vi "Pop.vi"(8 "error in (no error)":errorcluster, 11 "Signaller in":refnum<class "Signaller.lvclass">) -> (0 "error out":errorcluster, 2 "Has signal":bool, 3 "Signaller out":refnum<class "Signaller.lvclass">)   [LabVIEW 2018, in "Signaller.lvclass"]
uses:
  Signaller.lvclass
  Signaller.lvclass/Signaller.ctl
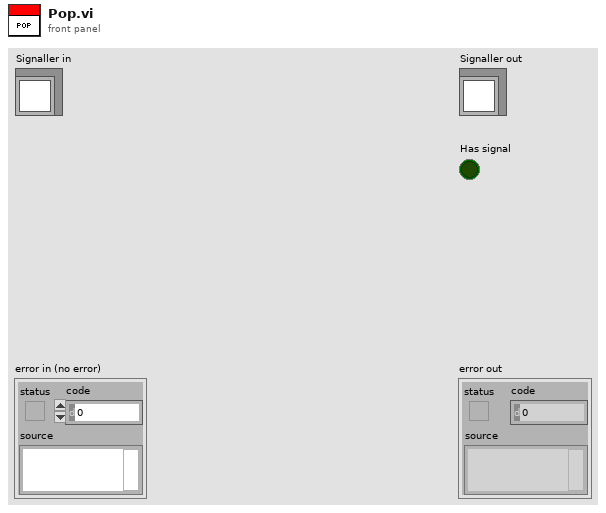
[diagram p1: front panel]
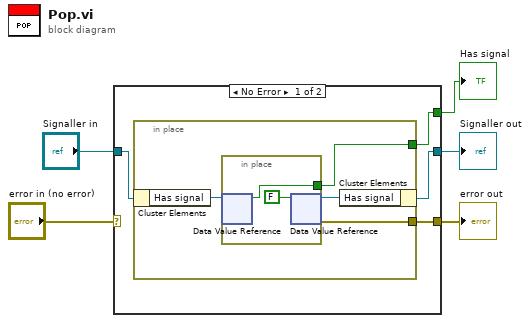
[diagram p0: block diagram]
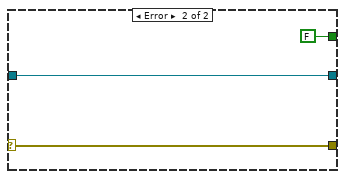
[diagram p2: hidden frame]
diagram:
  n1 = case shown="No Error" "error in (no error)" {
    selector: "error in (no error)" -> [_ w17]
    tunnel: [w6 w17] -> w4
    tunnel: [w8 w18] -> w2
    tunnel: "Signaller in" -> [w9 w18]
    tunnel: [w7 FALSE ("Has signal")] -> w1
    frame No Error {
      n2 = in-place {
        in-place-border: [w12] -> w7
        in-place-border: [w11] -> w6
        n3 = in-place-cluster #1(w9) -> ("Has signal"=w13:refnum<data-value>)
        n4 = in-place {
          in-place-border: [w14] -> w12
          n5 = in-place-dvr #2(w13) -> (w14:bool)  [unwired: 1 out]
          n6 = in-place-dvr #2(FALSE ("data value")) -> (w10:refnum<data-value>, w11:errorcluster)
        }
        n7 = in-place-cluster #1("Has signal"=w10) -> (w8:refnum<class "Signaller.lvclass">)
      }
    }
    frame Error {
    }
  }
  "error out" <- w4
  "Signaller out" <- w2
  "Has signal" <- w1
